vi "Test Helper Loop.vi"(8 "error in (no error)":errorcluster, 11 "Helper Loop Test In":refnum<class "Helper Loop Test.lvclass">) -> (0 "error out":errorcluster, 3 "Helper Loop Test Out":refnum<class "Helper Loop Test.lvclass">)   [LabVIEW 2020, in "Helper Loop Test.lvclass"]
uses:
  Helper Loop Test.lvclass
  C:/Program Files (x86)/National Instruments/LabVIEW 2020/vi.lib/Astemes/LUnit/Test Case.lvclass
  source/Framework Test Suite/Mock Process/Mock Process.lvclass
  C:/Git/astemes-triarc-framework/source/Framework/Process/Process.lvclass
  source/Framework/Process/Process.lvclass/Process.ctl
  <vilib>/Astemes/LUnit/Test Case.lvclass/Test Case.ctl
  940a0d52-585f-4e02-8690-06099146145a.vi
  source/Framework/Process/Public/Lifecycle/Get Lifecycle State.vi
  source/Framework/Broadcast Event Helpers/Execution timer.vi
  <vilib>/Astemes/LUnit/Palette/Pass.vi
  <vilib>/Astemes/LUnit/Palette/Fail.vi
  <vilib>/Astemes/LUnit/Compare Variants.vi
  <vilib>/Astemes/LUnit/Describe Comparison.vi
  <vilib>/Astemes/LUnit/Set Assertion Type.vi
  source/Framework/Process/Private/SubVIs/Wait for finish.vi
  source/Framework/Process/Private/SubVIs/Set Lifecycle State.vi
  source/Framework/Process/Protected/Messaging/Send Message.vi
  <vilib>/Utility/error.llb/Clear Errors.vi
  <vilib>/Astemes/LUnit/Add test result.vi
  <vilib>/Astemes/LUnit/Variant to string.vi
  source/Framework/Process/Private/SubVIs/Handle Debug Data.vi
  <vilib>/Astemes/LUnit/LUnit Record Assertion Result.vi
  source/Framework/Logging/Log Debug.vi
  <vilib>/AdvancedString/1D String Array to Delimited String.vi
  <vilib>/Utility/High Resolution Relative Seconds.vi
  <vilib>/Astemes/LUnit/LUnit Aggregate Assertion Results.vi
  <vilib>/Astemes/LUnit/Method Result/LUnit Merge Status.vi
  <vilib>/Astemes/LUnit/LUnit Concatenate result strings.vi
  <vilib>/Utility/error.llb/Error Cluster From Error Code.vi
  source/Framework/Broadcast Event Helpers/Dequeue Broadcast Message.vi
  <vilib>/Utility/Data Type/Get Type Information.vi
  <vilib>/Utility/LVClass/Get LV Class Name.vi
  source/Framework/Process/Public/Read Name.vi
  source/Framework/Process/Process.lvclass
  Helper Loop Test.lvclass/Helper Loop Test.ctl
  <vilib>/Astemes/LUnit/Test Case.lvclass
  source/Framework/Broadcast Event Helpers/Broadcast Event Helpers.lvlib
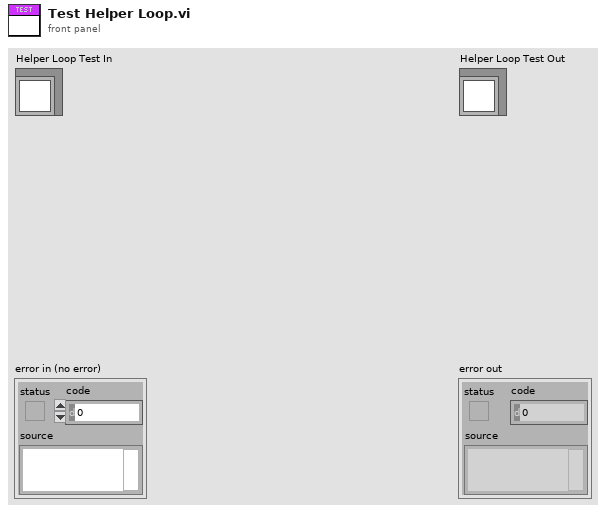
[diagram p1: front panel]
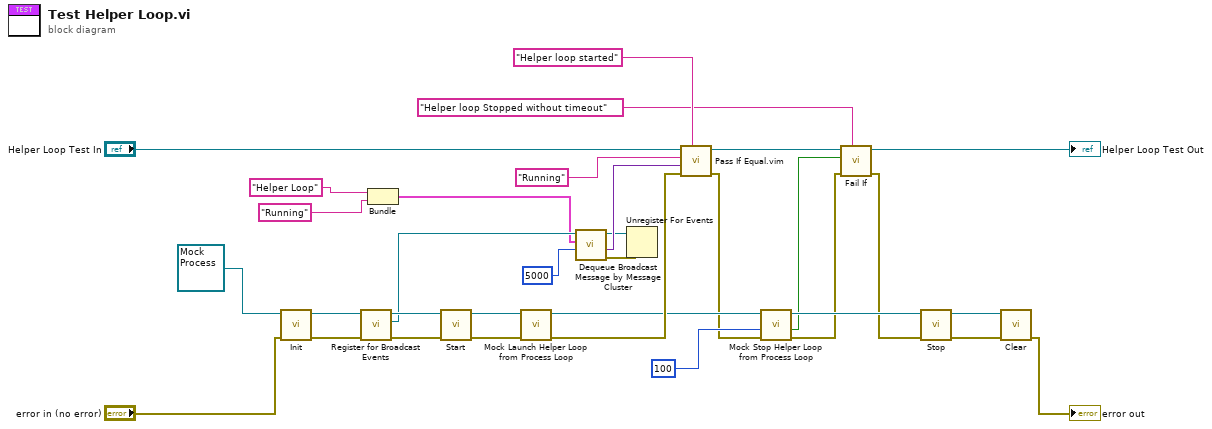
[diagram p0: block diagram]
diagram:
  n1 = call-dynamic "Init.vi"("error in (no error)"="error in (no error)", "Mock Process In"=refnum<class "Mock Process.lvclass"> refnum) -> ("error out"=w31:errorcluster, "Mock Process Out"=w32:refnum<class "Mock Process.lvclass">)  [unwired: 8 in]
  n2 = call "Register for Broadcast Events.vi"("error in (no error)"=w31, "Process In"=w32) -> ("error out"=w29:errorcluster, "Event Registration Refnum Out"=w6:refnum<event-registration>, "Process Out"=w30:refnum<class "Mock Process.lvclass">)  [unwired: 7 in]
  n3 = Bundle("y"="Helper Loop", "Description"="Running") -> (w1:cluster{"y":string, "Description":string})  [unwired: 1 in]
  n4 = call "Start.vi"("error in (no error)"=w29, "Process In"=w30) -> ("error out"=w27:errorcluster, "Process Out"=w28:refnum<class "Mock Process.lvclass">)  [unwired: 7 in, 1 out]
  n5 = call "Mock Launch Helper Loop from Process Loop.vi"("error in (no error)"=w27, "Mock Process in"=w28) -> ("error out"=w18:errorcluster, "Mock Process out"=w17:refnum<class "Mock Process.lvclass">)  [unwired: 8 in]
  n6 = call "Dequeue Broadcast Message by Message Cluster.vi"("Timeout (-1)"=5000, "Message"=w1, "Event Registration Refnum"=w6) -> ("error out"=w5:errorcluster, "Message Data"=w7:variant, "Event Registration Refnum Out"=w4:refnum<event-registration>)  [unwired: 4 in, 2 out]
  n7 = Unregister For Events(event registration refnum=w4, error in=w5) -> ()  [unwired: 1 out]
  n8 = call "Pass If Equal.vim"("Description"="Helper loop started", "error in (no error)"=w18, "Actual"=w7, "Expected"="Running", "LUnit Test Case In"="Helper Loop Test In") -> ("error out"=w15:errorcluster, "LUnit Test Case Out"=w23:refnum<class "Helper Loop Test.lvclass">)  [unwired: 5 in]
  n9 = call "Mock Stop Helper Loop from Process Loop.vi"("error in (no error)"=w15, "timeout in ms (-1)"=100, "Mock Process in"=w17) -> ("error out"=w12:errorcluster, "timed out?"=w14:bool, "Mock Process out"=w26:refnum<class "Mock Process.lvclass">)  [unwired: 6 in]
  n10 = call <vilib>:"Fail If.vi"("Description"="Helper loop Stopped without timeout", "error in (no error)"=w12, "Fail?"=w14, "LUnit Test Case In"=w23) -> ("error out"=w11:errorcluster, "LUnit Test Case Out"=→"Helper Loop Test Out":refnum<class "Helper Loop Test.lvclass">)  [unwired: 6 in]
  n11 = call "Stop.vi"("error in (no error)"=w11, "Process In"=w26) -> ("error out"=w25:errorcluster, "Process Out"=w10:refnum<class "Mock Process.lvclass">)  [unwired: 7 in, 1 out]
  n12 = call-dynamic "Clear.vi"("error in (no error)"=w25, "Mock Process In"=w10) -> ("error out"=→"error out":errorcluster)  [unwired: 9 in]
